vi "Identifier.vi"(8 "error in (no error)":errorcluster, 10 "Instrument Identifier":string, 11 "HSU MCU V2 in":refnum<class "HSU MCU V2.lvclass">) -> (0 "error out":errorcluster, 3 "HSU MCU V2 out":refnum<class "HSU MCU V2.lvclass">)   [LabVIEW 2024, in "HSU MCU V2.lvclass"]
uses:
  HSU MCU V2.lvclass
  HSU MCU V2.lvclass/HSU MCU V2.ctl
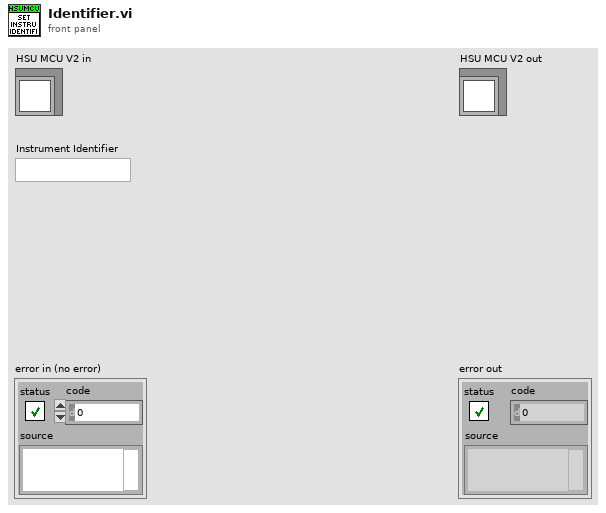
[diagram p1: front panel]
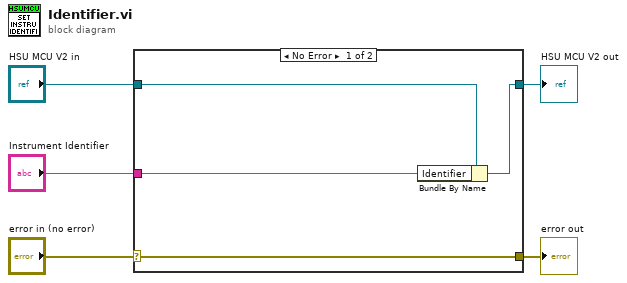
[diagram p0: block diagram]
diagram:
  n1 = case shown="No Error" "error in (no error)" {
    selector: "error in (no error)" -> [w9 w10]
    tunnel: [w9 w10] -> w4
    tunnel: [w7 w11] -> w2
    tunnel: "HSU MCU V2 in" -> [w8 w11]
    tunnel: "Instrument Identifier" -> [w6 _]
    frame No Error {
      n2 = Bundle By Name(cluster=w8, "Identifier"=w6) -> (w7:refnum<class "HSU MCU V2.lvclass">)
    }
    frame Error {
    }
  }
  "error out" <- w4
  "HSU MCU V2 out" <- w2
